vi "Server.vi"() -> ()   [LabVIEW 2025]
panel:
  out "Waveform Chart":dbl(graph)
  out "Alarm Message":string
  out "Alarm LED":bool
  out "Max Temp":dbl
  out "Min Temp":dbl
  out "Moving Avg":dbl
  out "Current Temp":dbl
  in  "Noise Amplitude":dbl=2.0
  in  "Low Threshold":dbl=15.0
  in  "High Threshold":dbl=30.0
  in  "Sample Period (ms)":dbl=500.0
  in  "Stop":bool
  in  "Start":bool
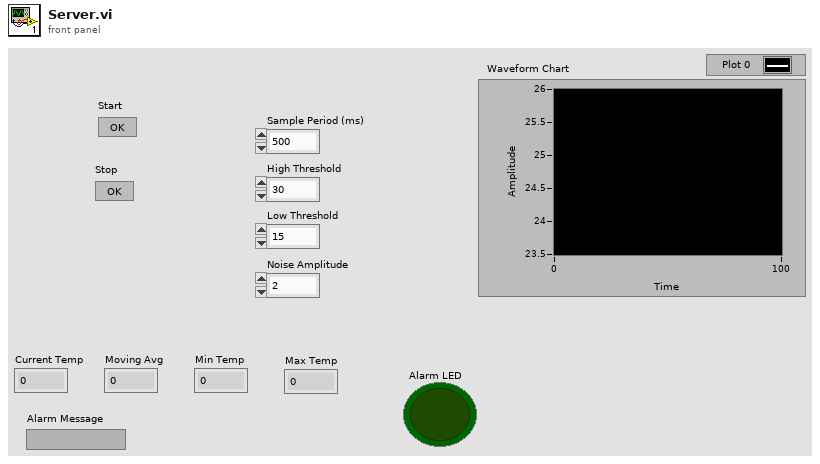
[diagram p1: front panel]
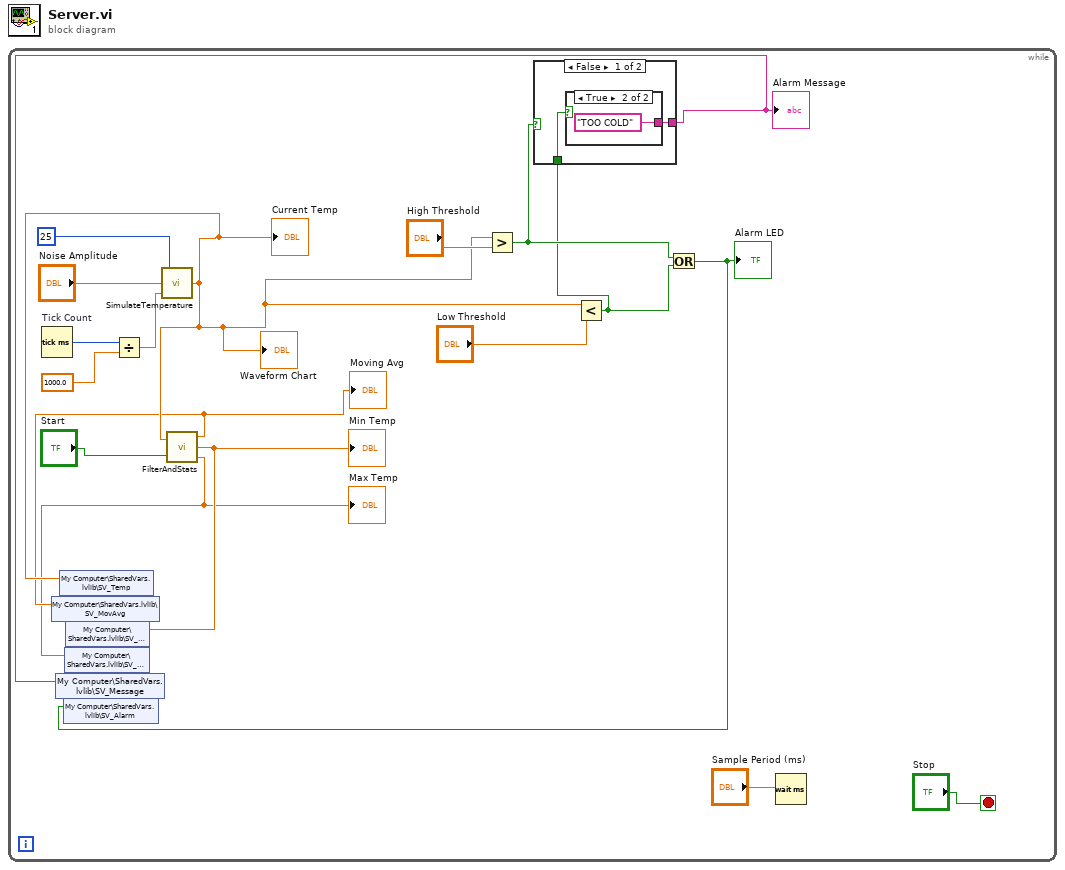
[diagram p0: block diagram]
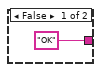
[diagram p2: hidden frame]
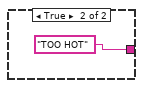
[diagram p3: hidden frame]
diagram:
  n1 = while {
    stop <- "Stop" stop-if-true
    n2 = Tick Count (ms) "Tick Count"() -> (millisecond timer value=w14:u32)
    n3 = Divide(x=w14, y=1000.0) -> (x/y=w12:dbl)
    n4 = call "SimulateTemperature.vi"("TimeSeconds"=w12, "NoiseAmp"="Noise Amplitude", "BaseTemp"=25) -> ("Temp Out"=w6:dbl)
    "Current Temp" <- w6
    "Waveform Chart" <- w6
    n5 = shared-variable "My Computer\\SharedVars.lvlib\\SV_Temp"(w6) -> ()  [unwired: 1 in, 1 out]
    n6 = call "FilterAndStats.vi"("TempIn"=w6, "Reset"="Start") -> ("MovAvg"=w5:dbl, "MinOut"=w4:dbl, "MaxOut"=w3:dbl)
    "Moving Avg" <- w5
    "Min Temp" <- w4
    "Max Temp" <- w3
    n7 = shared-variable "My Computer\\SharedVars.lvlib\\SV_MovAvg"(w5) -> ()  [unwired: 1 in, 1 out]
    n8 = shared-variable "My Computer\\SharedVars.lvlib\\SV_Max"(w3) -> ()  [unwired: 1 in, 1 out]
    n9 = shared-variable "My Computer\\SharedVars.lvlib\\SV_Min"(w4) -> ()  [unwired: 1 in, 1 out]
    n10 = Greater?(x=w6, y="High Threshold") -> (0:w8:bool)
    n11 = Less?(x=w6, y="Low Threshold") -> (x < y?=w7:bool)
    n12 = case shown="False" w8 {
      tunnel: w7 -> [w20 _]
      tunnel: [w19 "TOO HOT"] -> w2
      frame False {
        n13 = case shown="True" w20 {
          tunnel: ["OK" "TOO COLD"] -> w19
          frame False {
          }
          frame True {
          }
        }
      }
      frame True {
      }
    }
    "Alarm Message" <- w2
    n14 = shared-variable "My Computer\\SharedVars.lvlib\\SV_Message"(w2) -> ()  [unwired: 1 in, 1 out]
    n15 = Or(x=w8, y=w7) -> (x .or. y?=w1:bool)
    "Alarm LED" <- w1
    n16 = shared-variable "My Computer\\SharedVars.lvlib\\SV_Alarm"(w1) -> ()  [unwired: 1 in, 1 out]
    n17 = Wait (ms)(milliseconds to wait="Sample Period (ms)") -> ()  [unwired: 1 out]
  }
